vi "ADIS16448 Open.vi"(8 "error in":errorcluster, 9 "Initial Calibration Time (sec)":u32=4, 10 "Sychronous Process VI":T1, 11 "Hardware Config":T3={"SPI Clock Rate (Hz)"=1000000.0, "IMU SPI Mode (3)"=enum."Mode 3 (Clk Idle High,Sample on Trailing)", "IMU Reset Pin"=enum."DIO MXP 8", "IMU SPI Bus"=enum."SPI MXP", "IMU Data Ready Pin"=enum."DIO MXP 0", "Stall Config"={"Pow2BytesPerRead"=255, "StallTicks"=1000, "CsToSclkTicks"=100}, "IMU Status LED Pin"=enum."DIO MXP 9"}) -> (0 "error out":errorcluster, 3 "ADIS16448DevRef":T2={"DevStatus"={"status"=FALSE, "code"=0, "source"=""}, "Hardware Config"={"SPI Clock Rate (Hz)"=1000000.0, "IMU SPI Mode (3)"=enum."Mode 3 (Clk Idle High,Sample on Trailing)", "IMU Reset Pin"=enum."SPI Port CS2", "IMU SPI Bus"=enum."SPI On-Board, CS0", "IMU Data Ready Pin"=enum."SPI Port CS1", "Stall Config"={"Pow2BytesPerRead"=255, "StallTicks"=640, "CsToSclkTicks"=5}, "IMU Status LED Pin"=enum."DIO MXP 9"}, "Calibration Complete"=refnum, "Status FIFO"=refnum, "Last Value Reference"=refnum, "Sychronous Process VI"=refnum, "Cmd FIFO"=refnum, "Source"={"DevStatus"={"status"=FALSE, "code"=0, "source"=""}, "AnalogTriggerMode?"=FALSE, "DigitalMode"={"DIO Channel"=enum."Disabled"}, "AnalogTriggerMode"={"AnalogTriggerIndex"=enum."Trig 0", "OutputType"=enum."InWindow"}}, "Data FIFO"=refnum, "IMU Status LED Pin"=enum."DIO MXP 9", "Calibration Time"=5})   [LabVIEW 2019]
uses:
  Typedef/ADIS16448 Hardware Configuration.ctl
  <vilib>/Rock Robotics/WPI/SPI/WPI_SPIMode.ctl
  <vilib>/Rock Robotics/SystemInterfaces/DIO/FPGA_DIOChannel.ctl
  <vilib>/Rock Robotics/SystemInterfaces/spilib/spi_bus.ctl
  Typedef/ADIS16448 Device Reference.ctl
  Typedef/ADIS16448 Status.ctl
  Typedef/ADIS16448 Data.ctl
  Typedef/ADIS16448 Process.ctl
  Typedef/ADIS16448 Command Type.ctl
  <vilib>/Rock Robotics/SystemInterfaces/CounterEncoderSourceConvertion/FPGA_CounterEncoderSourceConvertionLVSourceType.ctl
  <vilib>/Rock Robotics/SystemInterfaces/DIO/FPGA_DIODigitalSourceChannel.ctl
  <vilib>/Rock Robotics/SystemInterfaces/AnalogTrigger/FPGA_AnalogTriggerIndex.ctl
  <vilib>/Rock Robotics/SystemInterfaces/AnalogTrigger/FPGA_AnalogTriggerOutType.ctl
  <vilib>/Rock Robotics/SystemInterfaces/NetworkCommunication/NetComm_UsageReport_ResourceType.ctl
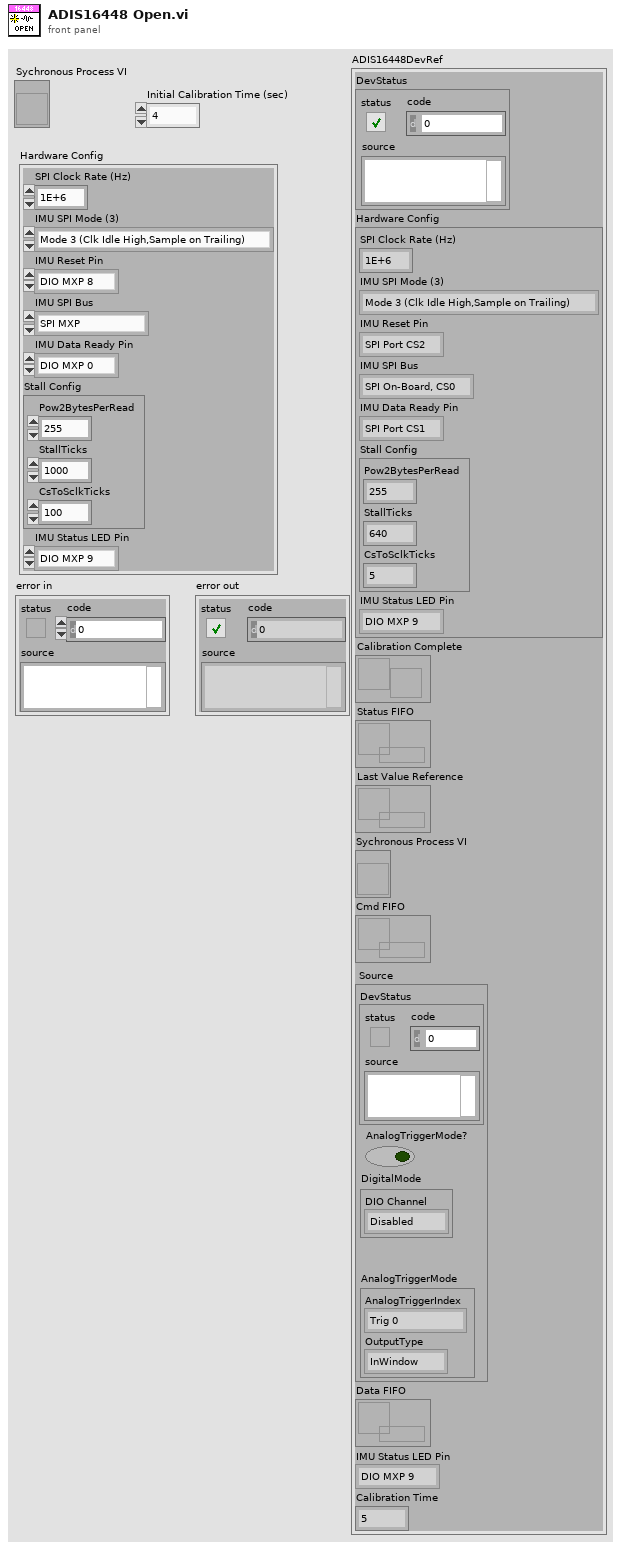
[diagram p1: front panel]
types:
  T1 = typedef "ADIS16448 Process.ctl" = refnum<vi>
  T2 = typedef "ADIS16448 Device Reference.ctl" = cluster{"DevStatus":errorcluster, "Hardware Config":T3, "Calibration Complete":refnum<notifier>, "Status FIFO":refnum<k33>, "Last Value Reference":refnum<data-value>, "Sychronous Process VI":T1, "Cmd FIFO":refnum<k33>, "Source":T7, "Data FIFO":refnum<k33>, "IMU Status LED Pin":T5, "Calibration Time":u32}
  T3 = typedef "ADIS16448 Hardware Configuration.ctl" = cluster{"SPI Clock Rate (Hz)":dbl, "IMU SPI Mode (3)":T4, "IMU Reset Pin":T5, "IMU SPI Bus":T6, "IMU Data Ready Pin":T5, "Stall Config":cluster{"Pow2BytesPerRead":u8, "StallTicks":u16, "CsToSclkTicks":u8}, "IMU Status LED Pin":T5}
  T4 = typedef "WPI_SPIMode.ctl" = enum16{"Mode 0 (Clk Idle Low,Sample on Leading)", "Mode 1 (Clk Idle Low,Sample on Trailing)", "Mode 2 (Clk Idle High,Sample on Leading)", "Mode 3 (Clk Idle High,Sample on Trailing)"}
  T5 = typedef "FPGA_DIOChannel.ctl" = enum8{"DIO 0", "DIO 1", "DIO 2", "DIO 3", "DIO 4", "DIO 5", "DIO 6", "DIO 7", "DIO 8", "DIO 9", "DIO MXP 0", "DIO MXP 1", "DIO MXP 2", "DIO MXP 3", "DIO MXP 4", "DIO MXP 5", "DIO MXP 6", "DIO MXP 7", "DIO MXP 8", "DIO MXP 9", "DIO MXP 10", "DIO MXP 11", "DIO MXP 12", "DIO MXP 13", "DIO MXP 14", "DIO MXP 15", "SPI Port CS1", "SPI Port CS2", "SPI Port CS3", "SPI Port MISO", "SPI Port MOSI", "Invalid"}
  T6 = typedef "spi_bus.ctl" = enum16{"SPI On-Board, CS0", "SPI On-Board, CS1", "SPI On-Board, CS2", "SPI On-Board, CS3", "SPI MXP", "Invalid"}
  T7 = typedef "FPGA_CounterEncoderSourceConvertionLVSourceType.ctl" = cluster{"DevStatus":errorcluster, "AnalogTriggerMode?":bool, "DigitalMode":cluster{"DIO Channel":T8}, "AnalogTriggerMode":cluster{"AnalogTriggerIndex":T9, "OutputType":T10}}
  T8 = typedef "FPGA_DIODigitalSourceChannel.ctl" = enum8{"DIO 0", "DIO 1", "DIO 2", "DIO 3", "DIO 4", "DIO 5", "DIO 6", "DIO 7", "DIO 8", "DIO 9", "DIO MXP 0", "DIO MXP 1", "DIO MXP 2", "DIO MXP 3", "DIO MXP 4", "DIO MXP 5", "DIO MXP 6", "DIO MXP 7", "DIO MXP 8", "DIO MXP 9", "DIO MXP 10", "DIO MXP 11", "DIO MXP 12", "DIO MXP 13", "DIO MXP 14", "DIO MXP 15", "SPI Port CS1", "SPI Port CS2", "SPI Port CS3", "SPI Port MISO", "SPI Port MOSI", "Disabled"}
  T9 = typedef "FPGA_AnalogTriggerIndex.ctl" = enum8{"Trig 0", "Trig 1", "Trig 2", "Trig 3", "Trig 4", "Trig 5", "Trig 6", "Trig 7", "Invalid"}
  T10 = typedef "FPGA_AnalogTriggerOutType.ctl" = enum16{"InWindow", "TriggerState", "Rising", "Falling"}
  T11 = typedef "ADIS16448 Command Type.ctl" = cluster{"Command":enum16{"None", "Reset", "Rewrite Config", "Start Recal", "Recalibrate", "Recal Complete", "Exit Auto SPI", "Start Auto SPI", "Configure Cal"}, "Data":u32}
  T12 = typedef "ADIS16448 Data.ctl" = cluster{"XAngle":dbl, "YAngle":dbl, "ZAngle":dbl}
  T13 = typedef "ADIS16448 Status.ctl" = cluster{"Calibrated?":bool, "IMU Detected?":bool}
  T14 = typedef "NetComm_UsageReport_ResourceType.ctl" = enum8{"Controller", "Module", "Language", "CANPlugin", "Accelerometer", "ADXL345", "AnalogChannel", "AnalogTrigger", "AnalogTriggerOutput", "CANJaguar", "Compressor", "Counter", "Dashboard", "DigitalInput", "DigitalOutput", "DriverStationCIO", "DriverStationEIO", "DriverStationLCD", "Encoder", "GearTooth", "Gyro", "I2C", "Framework", "Jaguar", "Joystick", "Kinect", "KinectStick", "PIDController", "Preferences", "PWM", "Relay", "RobotDrive", "SerialPort", "Servo", "Solenoid", "SPI", "Task", "Ultrasonic", "Victor", "Button", "Command", "AxisCamera", "PCVideoServer", "SmartDashboard", "Talon", "HiTechnicColorSensor", "HiTechnicAccel", "HiTechnicCompass", "SRF08", "AnalogOutput", "Victor SP", "Talon SRX", "CAN Talon SRX", "ADXL362 Accel", "ADXRS450 Gyro", "Rev SPARK", "Mindsensors SD540", "Digital Filter", "ADIS16448", "PDP", "PCM", "PigeonIMU", "Nidec Brushless", "CTRE CANifier", "CTRE TalonFX", "CTRE Future 1", "CTRE Future 2", "CTRE Future 3", "CTRE Future 4", "CTRE Future 5", "CTRE Future 6", "Linear Filter", "Xbox Controller", "USB Camera", "NavX", "Pixy", "Pixy2", "ScanseSweep", "Shuffleboard", "CAN", "Digilent DMC60", "PWM Victor SPX", "Rev SPARK MAX PWM", "Rev SPARK MAX CAN", "ADIS16470", "PIDController2", "ProfiledPIDController", "Kinematics", "Odometry", "Units", "Trapezoid Profile", "DutyCycle", "Addressable LEDs", "Fusion Venom"}
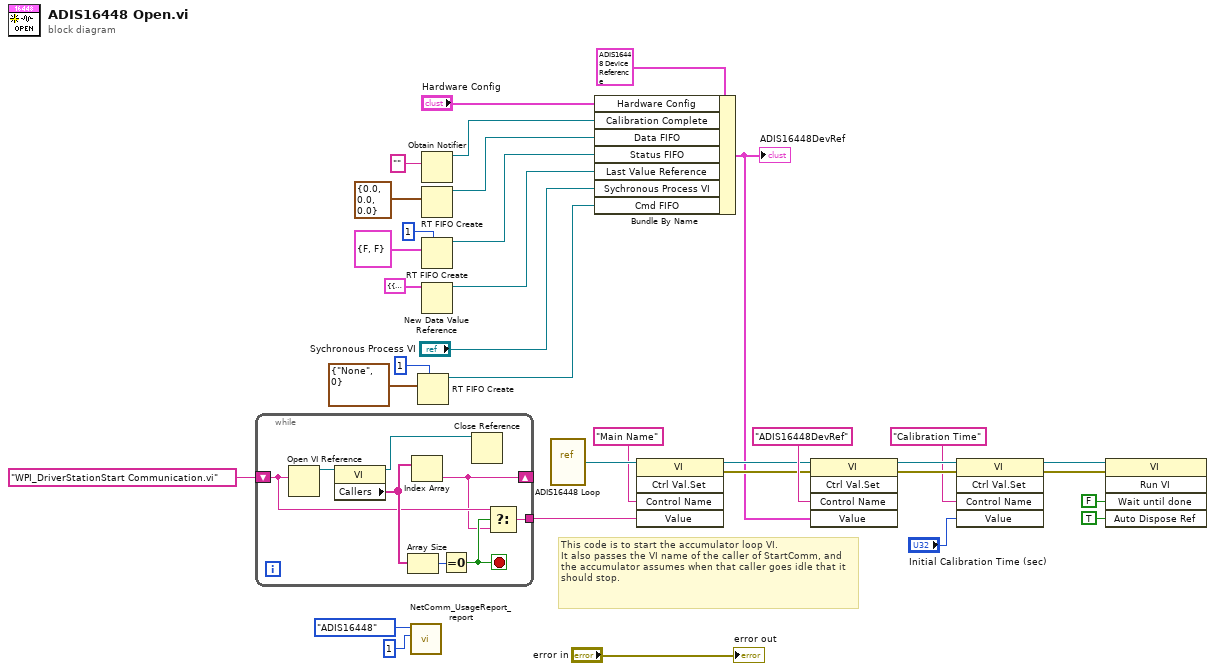
[diagram p0: block diagram]
diagram:
  # "This code is to start the accumulator loop VI.\nIt also passes the VI name of the caller of StartComm, and the accumulator assumes when that caller goes idle that it should stop."
  n1 = while {
    shift-right: [w37] -> _
    shift-left: "WPI_DriverStationStart Communication.vi" -> [w38]
    tunnel: [w36] -> w24
    stop <- w39 stop-if-true
    n2 = Open VI Reference(vi path=w38) -> (vi reference=w42:refnum<vi>)  [unwired: 1 in, 5 out]
    n3 = property class="VI"(reference=w42) -> (reference out=w35:refnum<vi>, "Callers"=w40:string[])  [unwired: 1 in, 1 out]
    n4 = Array Size(array=w40) -> (size(s)=w41:i32)
    n5 = Index Array(array=w40) -> (element=w37:string)  [unwired: 1 in]
    n6 = Equal To 0?(x=w41) -> (x = 0?=w39:bool)
    n7 = Close Reference(reference=w35) -> ()  [unwired: 1 in, 1 out]
    n8 = Select(t=w38, s=w39, f=w37) -> (s? t:f=w36:string)
  }
  n9 = call <vilib>:"NetComm_UsageReport_report.vi"("Instance Number"=u8 1, "Resource Type"=NetComm_UsageReport_ResourceType."ADIS16448") -> ()  [unwired: 10 in]
  n10 = RT FIFO Create(1:T11 {"Command"=enum."None", "Data"=0}, 4:u32 1 ("size (10)")) -> (8:w7:refnum<k33>)  [unwired: 6 in, 2 out]
  n11 = Obtain Notifier(notification data type="") -> (notifier out=w19:refnum<notifier>)  [unwired: 3 in, 2 out]
  n12 = RT FIFO Create(1:T12 {"XAngle"=0.0, "YAngle"=0.0, "ZAngle"=0.0}) -> (8:w14:refnum<k33>)  [unwired: 7 in, 2 out]
  n13 = RT FIFO Create(1:T13 {"Calibrated?"=FALSE, "IMU Detected?"=FALSE}, 4:u32 1 ("size (10)")) -> (8:w13:refnum<k33>)  [unwired: 6 in, 2 out]
  n14 = New Data Value Reference(data value=cluster{T12, T13} {{"XAngle"=0.0, "YAngle"=0.0, "ZAngle"=0.0}, {"Calibrated?"=FALSE, "IMU Detected?"=FALSE}} ("output cluster")) -> (data value reference=w11:refnum<data-value>)  [unwired: 1 in, 1 out]
  n15 = vi-ref "ADIS16448 Loop.vi"() -> (w26:refnum<vi>)
  n16 = Bundle By Name(cluster=T2 {"DevStatus"={"status"=FALSE, "code"=0, "source"=""}, "Hardware Config"={"SPI Clock Rate (Hz)"=1000000.0, "IMU SPI Mode (3)"=enum."Mode 3 (Clk Idle High,Sample on Trailing)", "IMU Reset Pin"=enum."SPI Port CS2", "IMU SPI Bus"=enum."SPI On-Board, CS0", "IMU Data Ready Pin"=enum."SPI Port CS1", "Stall Config"={"Pow2BytesPerRead"=255, "StallTicks"=640, "CsToSclkTicks"=5}, "IMU Status LED Pin"=enum."DIO MXP 9"}, "Calibration Complete"=refnum, "Status FIFO"=refnum, "Last Value Reference"=refnum, "Sychronous Process VI"=refnum, "Cmd FIFO"=refnum, "Source"={"DevStatus"={"status"=FALSE, "code"=0, "source"=""}, "AnalogTriggerMode?"=FALSE, "DigitalMode"={"DIO Channel"=enum."Disabled"}, "AnalogTriggerMode"={"AnalogTriggerIndex"=enum."Trig 0", "OutputType"=enum."InWindow"}}, "Data FIFO"=refnum, "IMU Status LED Pin"=enum."DIO MXP 9", "Calibration Time"=5} ("ADIS16470DevRef"), "Hardware Config"="Hardware Config", "Calibration Complete"=w19, "Data FIFO"=w14, "Status FIFO"=w13, "Last Value Reference"=w11, "Sychronous Process VI"="Sychronous Process VI", "Cmd FIFO"=w7) -> (w20:T2)
  "ADIS16448DevRef" <- w20
  n17 = invoke class="VI" method="Ctrl Val.Set"(reference=w26, "Control Name"="Main Name", "Value"=w24) -> (reference out=w23:refnum<vi>, error out=w28:errorcluster)  [unwired: 2 in, 3 out]
  n18 = invoke class="VI" method="Ctrl Val.Set"(reference=w23, error in=w28, "Control Name"="ADIS16448DevRef", "Value"=w20) -> (reference out=w6:refnum<vi>, error out=w5:errorcluster)  [unwired: 1 in, 3 out]
  n19 = invoke class="VI" method="Ctrl Val.Set"(reference=w6, error in=w5, "Control Name"="Calibration Time", "Value"="Initial Calibration Time (sec)") -> (reference out=w3:refnum<vi>, error out=w2:errorcluster)  [unwired: 1 in, 3 out]
  n20 = invoke class="VI" method="Run VI"(reference=w3, error in=w2, "Wait until done"=FALSE ("Wait Until Done"), "Auto Dispose Ref"=TRUE ("Auto Dispose Reference")) -> ()  [unwired: 1 in, 5 out]
  "error out" <- "error in"
